vi "Calculate MUX Values.vi"(8 "error in (no error)":errorcluster, 10 "Channels":i32[](array[ring]) items=["Channel A"=1, "Channel B"=2, "Channel C"=3, "Channel D"=4, "Channel E"=5, "Channel F"=6, "Channel G"=7, "Channel H"=8], 11 "VISA resource name":refnum<visa-resource-name>) -> (0 "error out":errorcluster, 2 "MUX Value":i32, 3 "VISA resource name out":refnum<visa-resource-name>)   [LabVIEW 2012, in "Quantum Composers 9000 Series.lvlib"]
doc: "This utility VI can be used to calculate the MUX value needed to multiplex multiple channels to an output."
uses:
  <instrlib>/Quantum Composers 9000 Series/Quantum Composers 9000 Series.lvlib
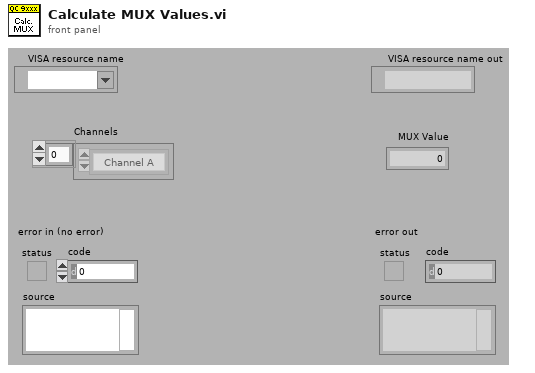
[diagram p1: front panel]
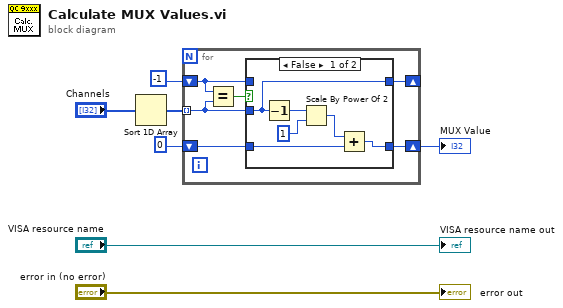
[diagram p0: block diagram]
diagram:
  n1 = Sort 1D Array(array="Channels") -> (sorted array=w5:i32[])
  n2 = for {
    shift-right: [w13] -> w6
    shift-left: 0 ("Chan MUX Value Out") -> [w12]
    tunnel: w5 -> [w9] mode=indexing
    shift-right: [w8] -> _
    shift-left: -1 ("Chan #") -> [w10]
    n3 = Equal?(x=w10, y=w9) -> (x = y?=w11:bool)
    n4 = case shown="False" w11 {
      tunnel: w9 -> [w14 _]
      tunnel: [w16 w20] -> w13
      tunnel: w12 -> [w15 w20]
      tunnel: w10 -> [_ w21]
      tunnel: [w14 w21] -> w8
      frame False {
        n5 = Decrement(x=w14) -> (x-1=w18:i32)
        n6 = Scale By Power Of 2(n=w18, x=1) -> (x*2^n=w17:i32)
        n7 = Add(x=w17, y=w15) -> (x+y=w16:i32)
      }
      frame True {
      }
    }
  }
  "MUX Value" <- w6
  "error out" <- "error in (no error)"
  "VISA resource name out" <- "VISA resource name"
